vi "temp bypass.vi"() -> ()   [LabVIEW 2016]
uses:
  new-h-nu-ixon/Emission filters.ctl
  new-h-nu-ixon/Filter wheel settings globals.vi
panel:
  out ".not. x?":bool
  in  "Emission filter wheel":T1
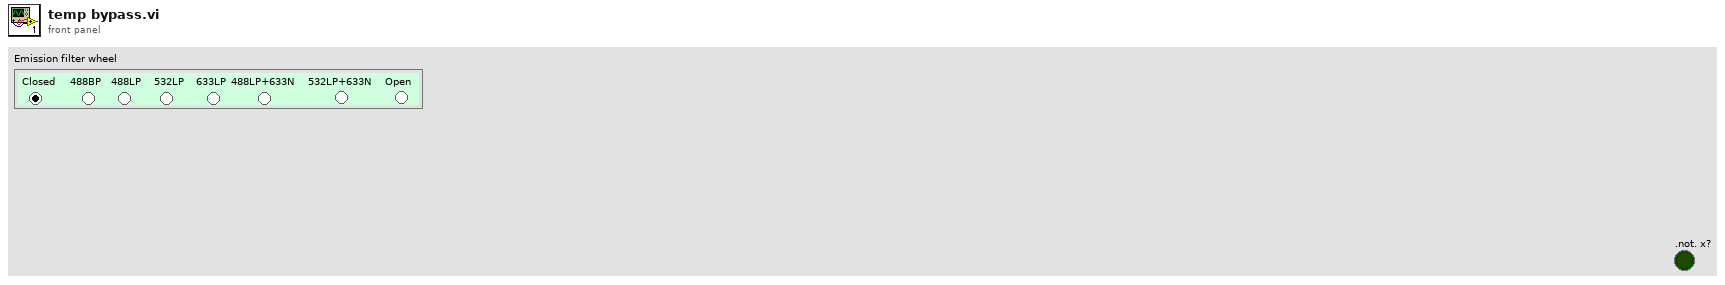
[diagram p1: front panel]
types:
  T1 = typedef "Emission filters.ctl" = enum32{" Closed ", " 488BP ", "488LP", "  532LP ", "633LP", "488LP+633N", "532LP+633N", "Open"}
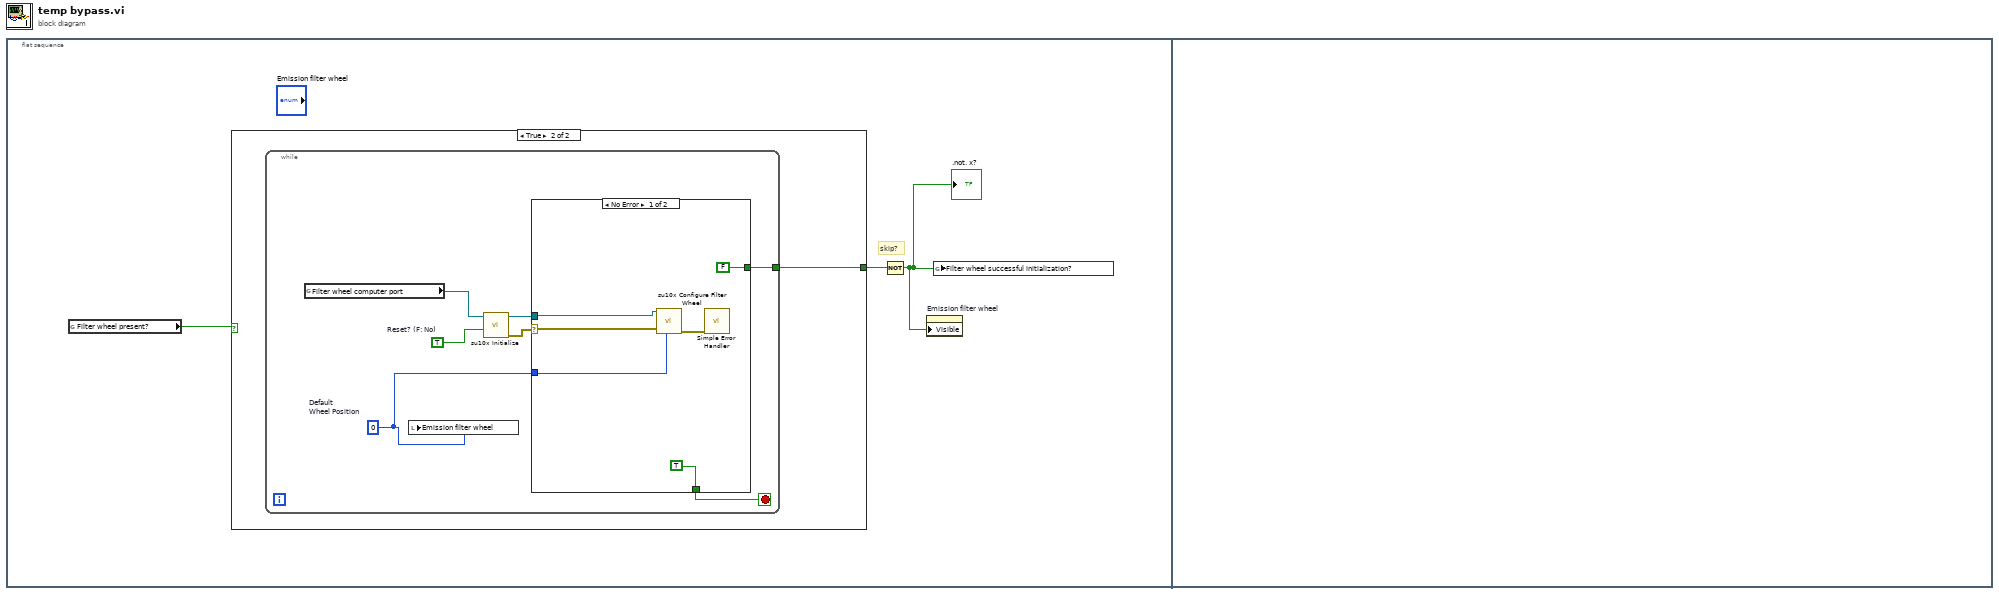
[diagram p0: block diagram]
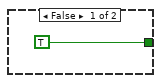
[diagram p2: hidden frame]
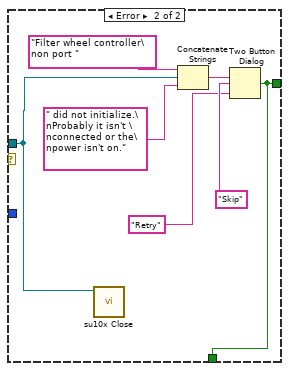
[diagram p3: hidden frame]
diagram:
  n1 = flat-sequence {
    frame #0 {
      # "skip?"
      n2 = global read "Filter wheel settings globals.vi" "Filter wheel present?"() -> (w1:bool)
      n3 = case shown="True" w1 {
        tunnel: [TRUE ("T button?") w5] -> w2
        frame False {
        }
        frame True {
          n4 = while {
            tunnel: [w7] -> w5
            stop <- w9 stop-if-true
            w6 = u8 0  # Default Wheel Position
            w11 = TRUE  # Reset? (F: No)
            n5 = global read "Filter wheel settings globals.vi" "Filter wheel computer port"() -> (w12:refnum<visa-resource-name>)
            n6 = local write "Emission filter wheel"(w6) -> ()
            n7 = call <instrlib>:"su10x Initialize.vi"("Reset? (F: No)"=w11, "VISA resource name"=w12) -> ("error out"=w10:errorcluster, "VISA resource name out"=w8:refnum<visa-resource-name>)  [unwired: 2 in, 6 out]
            n8 = case shown="No Error" w10 {
              selector: w10 -> [w17 _]
              tunnel: [TRUE w19] -> w9
              tunnel: w8 -> [w16 w20]
              tunnel: [FALSE ("T button?") w19] -> w7
              tunnel: w6 -> [w14 _]
              frame No Error {
                n9 = call <instrlib>:"su10x Configure Filter Wheel.vi"("Wheel Position (0)"=w14, "error in (no error)"=w17, "VISA resource name"=w16) -> ("error out"=w13:errorcluster)  [unwired: 2 in, 6 out]
                n10 = call <vilib>:"Simple Error Handler.vi"("error in (no error)"=w13) -> ()  [unwired: 1 in, 8 out]
              }
              frame Error {
                n11 = call <instrlib>:"su10x Close.vi"("VISA resource name"=w20) -> ()  [unwired: 1 in, 10 out]
                n12 = Concatenate Strings("Filter wheel controller\non port " ("string"), w20, " did not initialize.\nProbably it isn't \nconnected or the\npower isn't on." ("string")) -> (w25:string)
                n13 = Two Button Dialog(message=w25, 1:"Retry" ("F button name (\"Cancel\")"), 2:"Skip" ("T button name (\"OK\")")) -> (T button?=w19:bool)
              }
            }
          }
        }
      }
      n14 = Not(x=w2) -> (.not. x?=w3:bool)
      ".not. x?" <- w3
      n15 = property on="Emission filter wheel" class="RadioBtnsControl (strict)"("Visible"=w3) -> ()  [unwired: 2 in, 2 out]
      n16 = global write "Filter wheel settings globals.vi" "Filter wheel successful initialization?"(w3) -> ()
    }
    frame #1 {
    }
  }
